vi "price.vi"(8 "error in (no error)":errorcluster, 11 "Pepsi in":refnum<class "Pepsi.lvclass">) -> (0 "error out":errorcluster, 2 "price":dbl, 3 "Pepsi out":refnum<class "Pepsi.lvclass">)   [LabVIEW 2018, in "Pepsi.lvclass"]
uses:
  Pepsi.lvclass
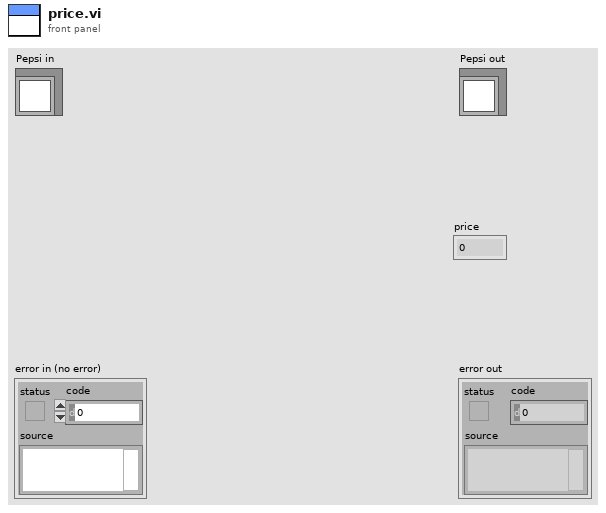
[diagram p1: front panel]
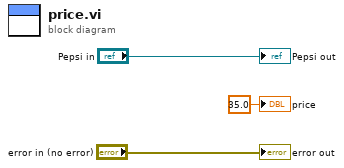
[diagram p0: block diagram]
diagram:
  "error out" <- "error in (no error)"
  "Pepsi out" <- "Pepsi in"
  "price" <- 35.0 ("price")
